vi "Normal to Hex String.vi"(1 "Normal In":string) -> (0 "Hex Out":string)   [LabVIEW 2014, in "StringConvert.lvlib"]
uses:
  StringConvert.lvlib
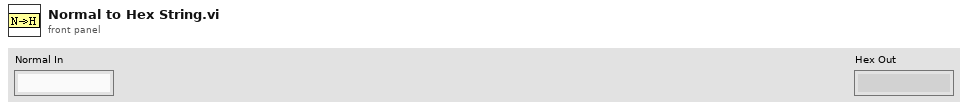
[diagram p1: front panel]
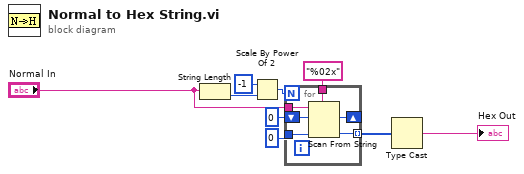
[diagram p0: block diagram]
diagram:
  n1 = String Length(string="Normal In") -> (length=w7:i32)
  n2 = Scale By Power Of 2(n=-1, x=w7) -> (x*2^n=w5:i32)
  n3 = for {
    N: w5 -> [_]
    shift-right: [w14] -> _
    shift-left: u32 0 -> [w15]
    tunnel: "Normal In" -> [w13]
    tunnel: u8 0 ("U8") -> [w12]
    tunnel: [w11] -> w3 mode=indexing
    tunnel: "%02x" ("format string") -> [w10]
    n4 = Scan From String(format string=w10, input string=w13, initial scan location=w15, default 1=w12) -> (offset past scan=w14:u32, output 1=w11:u8)  [unwired: 1 in, 2 out]
  }
  n5 = Type Cast(x=w3) -> (*(type *) &x=→"Hex Out":string)  [unwired: 1 out]
